vi "设置仪器参数命令解析.vi"(8 "error in (no error)":errorcluster caption="错误输入（无错误）", 11 "String输入":string) -> (0 "error out":errorcluster caption="错误输出", 3 "设置参数信息数组":string[][](array[string]))   [LabVIEW 2016, in "数据传输系统.lvlib"]
panel:
  out "大小":i32[](array[numeric])
  out "数组":string[](array[string])
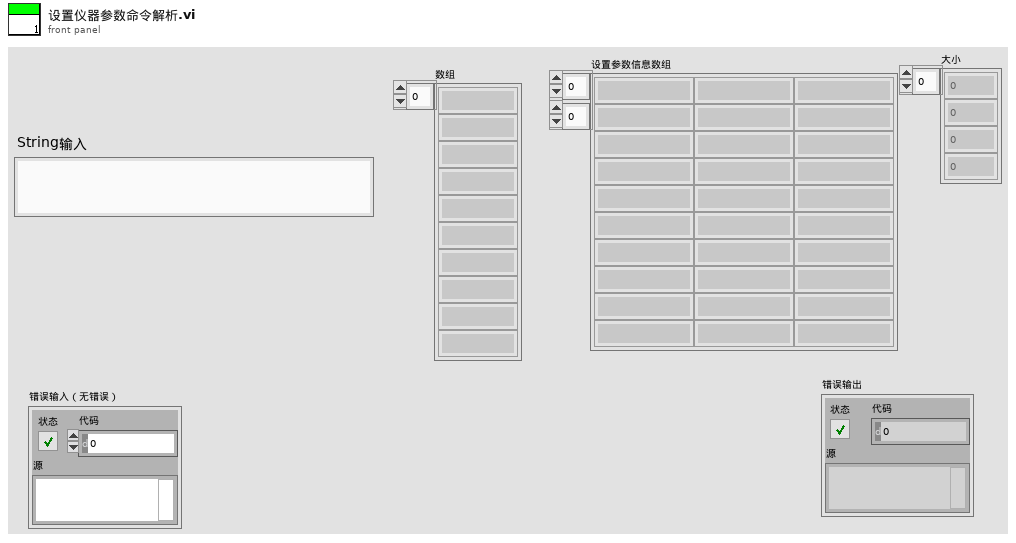
[diagram p1: front panel]
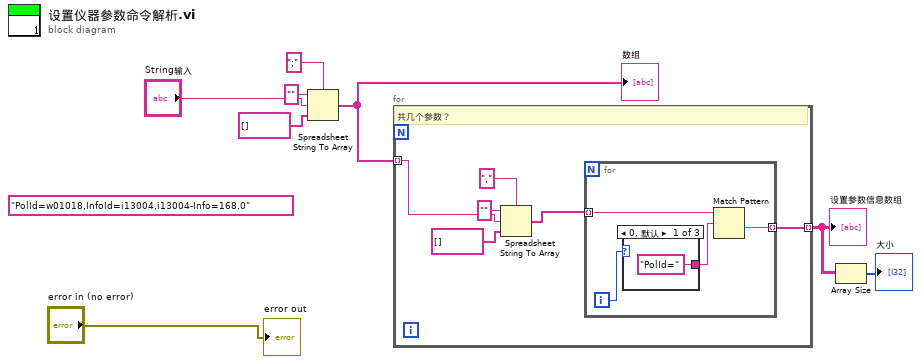
[diagram p0: block diagram]
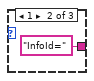
[diagram p2: hidden frame]
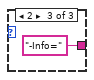
[diagram p3: hidden frame]
diagram:
  (unwired) "PolId=w01018,InfoId=i13004,i13004-Info=168.0"
  n1 = Spreadsheet String To Array(delimiter (Tab)=";" ("分隔符(Tab)"), format string="" ("格式字符串"), spreadsheet string="String输入", array type (2D Dbl)=string[] []) -> (array=w3:string[])
  "数组" <- w3
  n2 = for {
    tunnel: w3 -> [w11] mode=indexing
    tunnel: [w9] -> w1 mode=indexing
    # "共几个参数？"
    n3 = Spreadsheet String To Array(delimiter (Tab)="," ("分隔符(Tab)"), format string="" ("格式字符串"), spreadsheet string=w11, array type (2D Dbl)=string[] []) -> (array=w10:string[])
    n4 = for {
      tunnel: w10 -> [w18] mode=indexing
      tunnel: [w15] -> w9 mode=indexing
      i -> [w17]
      n5 = case shown="0, 默认" w17 {
        tunnel: ["PolId=" "InfoId=" "-Info="] -> w16
        frame 0, Default {
        }
        frame 1 {
        }
        frame 2 {
        }
      }
      n6 = Match Pattern(string=w18, regular expression=w16) -> (after substring=w15:string)  [unwired: 1 in, 3 out]
    }
  }
  "设置参数信息数组" <- w1
  n7 = Array Size(array=w1) -> (size(s)=→"大小":i32[])
  "error out" <- "error in (no error)"
